vi "WT300 Read Power Only.vi"(8 "Error In":errorcluster) -> (0 "Error Out":errorcluster)   [LabVIEW 2019]
uses:
  Trunk/Utility/Type Definitions/UTILITY Power Data.ctl
panel:
  out "Power Data":T1={"Current (A):Element 1"=236.2, "Current (A):Element 2"=17.749, "Power (W):Sigma"=4192.0, "Watt Hours (Wh):Sigma"=0.0, "Voltage (V):Element 2"=236.2, "Voltage (V):Element 1"=236.2, "Current Crest Factor:Element 1"=0.0, "Current Crest Factor:Element 2"=0.0, "Voltage Harmonic (%):Element 1"=0.0, "Voltage Harmonic (%):Element 2"=0.0, "Voltage Crest Factor:Element 1"=0.0, "Voltage Crest Factor:Element 2"=0.0, "Time:Element 1"=0.0, "Frequency (Hz):Element 1"=0.0, "Apparent Power (VA):Element 1"=0.0, "Apparent Power (VA):Element 2"=0.0, "Power Factor:Element 1"=0.0, "Power Factor:Element 2"=0.0, "Max Watt Hours"=0.0, "Voltage (V):Element 2 Avg"=0.0, "Voltage (V):Element 1 Avg"=0.0} {"Voltage (V):Element 1 Avg" format="%.3g"; "Voltage (V):Element 2 Avg" format="%.3g"; "Max Watt Hours" format="%.3g"; "Power Factor:Element 2" format="%.3g"; "Power Factor:Element 1" format="%.3g"; "Apparent Power (VA):Element 2" format="%.3g"; "Apparent Power (VA):Element 1" format="%.3g"; "Frequency (Hz):Element 1" format="%.3g"; "Time:Element 1" format="%.3g"; "Voltage Crest Factor:Element 2" format="%.3g"; "Voltage Crest Factor:Element 1" format="%.3g"; "Voltage Harmonic (%):Element 2" format="%.3g"; "Voltage Harmonic (%):Element 1" format="%.3g"; "Current Crest Factor:Element 2" format="%.3g"; "Current Crest Factor:Element 1" format="%.3g"; "Voltage (V):Element 1" format="%.3g"; "Voltage (V):Element 2" format="%.3g"; "Watt Hours (Wh):Sigma" format="%.3f"; "Power (W):Sigma" format="%.3g"; "Current (A):Element 2" format="%.3e"; "Current (A):Element 1" format="%.3e"}
  in  "Timeout (10000 ms)":i32=1000
  out "Integrate Status List":bool[][](array[boolean])
  in  "Range Configuration (True)":bool[](array[boolean])=[FALSE, FALSE, FALSE, FALSE, FALSE, TRUE, TRUE, TRUE, TRUE, TRUE, TRUE, TRUE, FALSE]
  in  "Manual Range (20 <10> A)":dbl(ring)=10.0 items=["5m <2.5m>"=0.0025, "10m <5m>"=0.005, "20m <10m>"=0.01, "50m <25m>"=0.025, "100m <50m>"=0.05, "200m <100m>"=0.1, "500m <250m>"=0.25, "1 <500m>"=0.5, "2 <1>"=1.0, "5 <2.5>"=2.5, "10 <5>"=5.0, "20 <10>"=10.0, "40 <20>"=20.0]
  in  "Update Rate (250m s)":dbl(ring)=0.5 items=["100m"=0.1, "250m"=0.25, "500m"=0.5, "1"=1.0, "2"=2.0, "5"=5.0]
  in  "Enable Auto Range (F: Disable)":bool=TRUE
  out "Yokogawa Data":string[][](array[string])
  out "Header File":string[][](array[string])
  in  "VISA Input":refnum<visa-resource-name>
  in  "stop":bool
  # "5m <2.5m> A"
  # "10m <5m> A"
  # "20m <10m> A"
  # "50m <25m> A"
  # "100m <50m> A"
  # "200m <100m> A"
  # "500m <250m> A"
  # "1 <500m> A"
  # "2 <1> A"
  # "5 <2.5> A"
  # "10 <5> A"
  # "20 <10> A"
  # "40 <20> A"
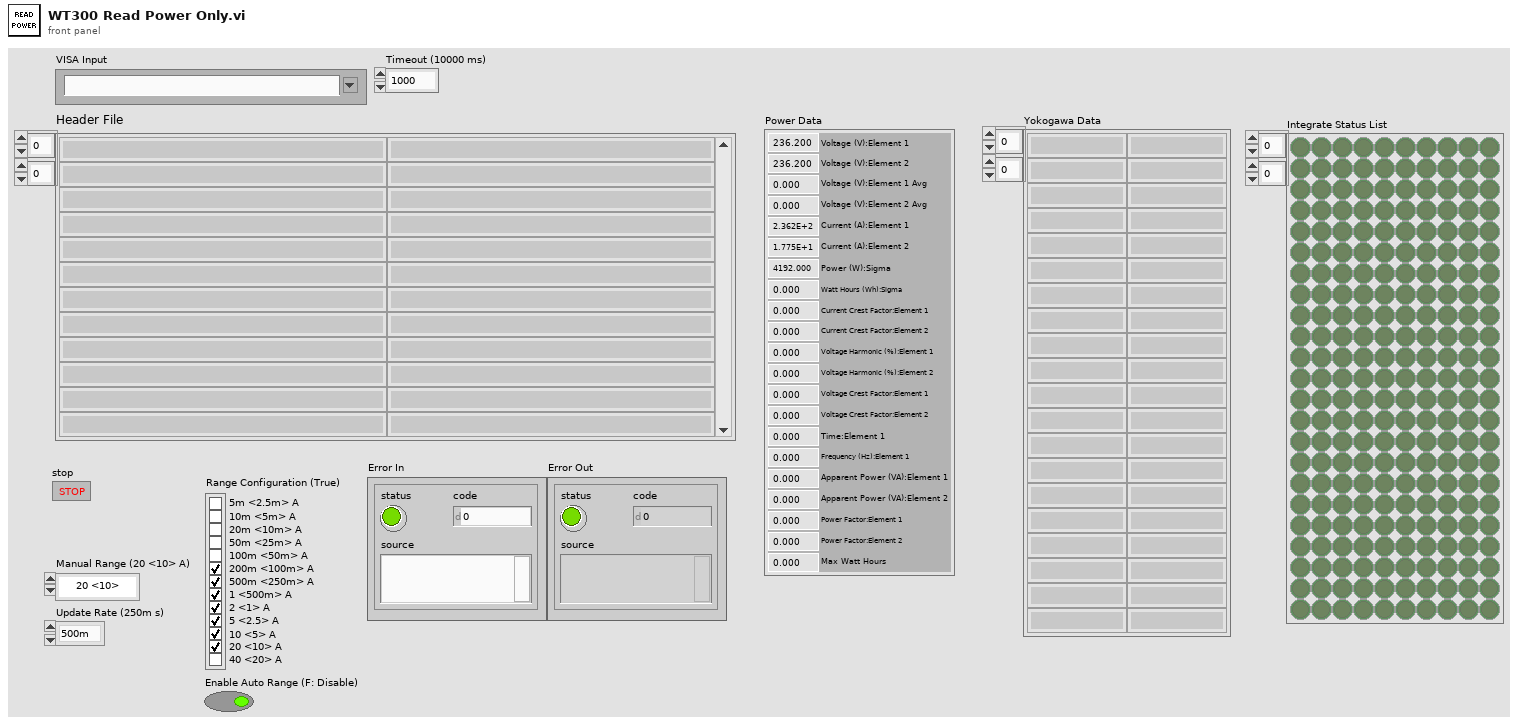
[diagram p1: front panel]
types:
  T1 = typedef "UTILITY Power Data.ctl" = cluster{"Current (A):Element 1":dbl, "Current (A):Element 2":dbl, "Power (W):Sigma":dbl, "Watt Hours (Wh):Sigma":dbl, "Voltage (V):Element 2":dbl, "Voltage (V):Element 1":dbl, "Current Crest Factor:Element 1":dbl, "Current Crest Factor:Element 2":dbl, "Voltage Harmonic (%):Element 1":dbl, "Voltage Harmonic (%):Element 2":dbl, "Voltage Crest Factor:Element 1":dbl, "Voltage Crest Factor:Element 2":dbl, "Time:Element 1":dbl, "Frequency (Hz):Element 1":dbl, "Apparent Power (VA):Element 1":dbl, "Apparent Power (VA):Element 2":dbl, "Power Factor:Element 1":dbl, "Power Factor:Element 2":dbl, "Max Watt Hours":dbl, "Voltage (V):Element 2 Avg":dbl, "Voltage (V):Element 1 Avg":dbl}
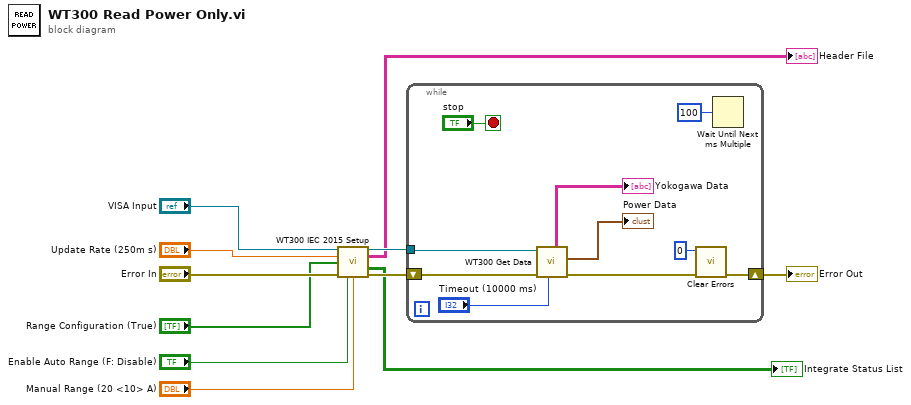
[diagram p0: block diagram]
diagram:
  n1 = call "WT300 IEC 2015 Setup.vi"("VISA Input"="VISA Input", "Update Rate (250m s)"="Update Rate (250m s)", "Range Configuration (True)"="Range Configuration (True)", "error in (no error)"="Error In", "Enable Auto Range (F: Disable)"="Enable Auto Range (F: Disable)", "Manual Range (20 <10> A)"="Manual Range (20 <10> A)") -> ("VISA Output"=w11:refnum<visa-resource-name>, "Header File"=→"Header File":string[][], "Integrate Status List"=→"Integrate Status List":bool[][], "error out"=w6:errorcluster)  [unwired: 5 in, 1 out]
  n2 = while {
    tunnel: w11 -> [w20]
    shift-right: [w15] -> w7
    shift-left: w6 -> [w21]
    stop <- "stop" stop-if-true
    n3 = call "WT300 Get Data.vi"("Timeout (10000 ms)"="Timeout (10000 ms)", "error in (no error)"=w21, "VISA resource name"=w20) -> ("error out"=w16:errorcluster, "Power Data"=→"Power Data":T1, "Yokogawa Data"=→"Yokogawa Data":string[][])  [unwired: 3 in, 3 out]
    n4 = call <vilib>:"Clear Errors.vi"("error in (no error)"=w16, "specific error code to clear (0: all)"=0) -> ("error out"=w15:errorcluster)  [unwired: 4 in, 1 out]
    n5 = Wait Until Next ms Multiple(millisecond multiple=u32 100) -> ()  [unwired: 1 out]
  }
  "Error Out" <- w7
